vi "PAT Device Software.vi"() -> ()   [LabVIEW 2018]
uses:
  <vilib>/Analysis/baseanly.llb/Mean (DBL).vi
  <vilib>/DAQmx/miscellaneous.llb/DAQmx Fill In Error Info.vi
  <vilib>/DAQmx/read.llb/DAQmx Read (Analog 1D Wfm NChan NSamp).vi
  <vilib>/DAQmx/configure/task.llb/DAQmx Configure Logging (TDMS).vi
  <vilib>/DAQmx/configure/timing.llb/DAQmx Timing (Sample Clock).vi
  <vilib>/DAQmx/create/channels.llb/DAQmx Create Channel (AI-Voltage-Basic).vi
  <vilib>/Instr/_visa.llb/VISA Configure Serial Port (Instr).vi
  <vilib>/Analysis/NI_AALBase.lvlib
panel:
  in  "Relay Comport":refnum<visa-resource-name>="COM7"
  in  "Boolean":bool
  in  "TDMS File Path":path
  in  "Motor Speed Control":dbl=5.0
  in  "Sample Rate":i32=10
  in  "CV2 Input Channel":tag="Dev1/ai0"
  in  "CV1 Input Channel":tag="Dev1/ai1"
  in  "TA Channel":tag="Dev1/ai6"
  in  "RHA Channel":tag="Dev1/ai7"
  in  "P1 Channel":tag="Dev1/ai5"
  out "Stop Test":bool=TRUE
  out "Is PAT Test?":bool=TRUE
  in  "Test Begin":bool
  out "Test Duration":i32
  out "Current Test":string
  out "Test Underway":i32
  out "Number of tests":i32
  out "Test List":i16[](array[numeric])
  out "error out 3":errorcluster
  in  "error in 2":errorcluster
  out "error out 2":errorcluster
  in  "error in":errorcluster
  out "error out":errorcluster
  in  "error in (no error)":errorcluster
  in  "Tab Control":enum32{"PAT Test", "Manual Control"}(tab)
  out "PAT Test Readings":T1 {"B40 S" scale=0.0..100.0; "B15 S" scale=0.0..100.0; "Ex70 S" scale=0.0..100.0; "Ex30 S" scale=0.0..100.0; "In70 S" scale=0.0..100.0; "In30 S" scale=0.0..100.0}
  out "Status":string="Status"
  out "Time":string="Time (s)"
  out "Limit":string="Limit"
  out "Comp":string="Comp"
  out "Units":string="Units"
  out "Measured":string="Measured"
  out "Test Name":string="Test Name"
  out "String 22":string="-0.8"
  out "String 15":string=">="
  out "String 8":string="in H2O"
  out "String":string="Inhalation (30lpm)"
  out "String 24":string="0.8"
  out "String 17":string="<="
  out "String 10":string="in H2O"
  out "String 3":string="Exhalation (30lpm)"
  out "String 23":string="-2.0"
  out "String 16":string=">="
  out "String 9":string="in H2O"
  out "String 2":string="Inhalation (70lpm)"
  out "String 26":string="26"
  out "String 19":string=">="
  out "String 12":string="% O2"
  out "String 5":string="Breathing (15kft)"
  out "String 25":string="2.0"
  out "String 18":string="<="
  out "String 11":string="in H2O"
  out "String 4":string="Exhalation (70lpm)"
  out "String 27":string="89"
  out "String 20":string=">="
  out "String 13":string="% O2"
  out "String 6":string="Breathing (40kft)"
  in  "Start PAT Test":bool
  in  "Stop PAT Test":bool
  out "Test Status:":string
  in  "Results File Location:":path=path "X:/Working/Finn Sowerbutts/Aerox/PAT/CDR Files/PAT Device Software/Test Reports"
  in  "PAT Test Settings":T2={"Test Date:"="", "Test Time:"="", "Pull Test Date:"="", "Operator:"="", "Production Order No.:"="", "Production Lot:"="", "No. Masks in Lot:"="", "Comments:"="", "Array"=[TRUE, TRUE, TRUE, TRUE, TRUE, TRUE], "Test Parameters:"=enum."Quick Test", "Facepiece Leakage"=0.0}
  out "Test Mode:":string[][](table)
  in  "Preset Directory:":path=path "X:/Working/Finn Sowerbutts/Aerox/PAT/CDR Files/PAT Device Software/Presets"
  in  "MC Fields":T3
  in  "MC Instrumentation":T4
  in  "Start Custom Test":bool
  in  "Stop Custom Test":bool
  # "ccm"
  # "s"
  # "Pamb"
  # "Tamb"
  # "Hamb"
  # "in H2O"
  # "°C"
  # "%"
  # "F2"
  # "ccm"
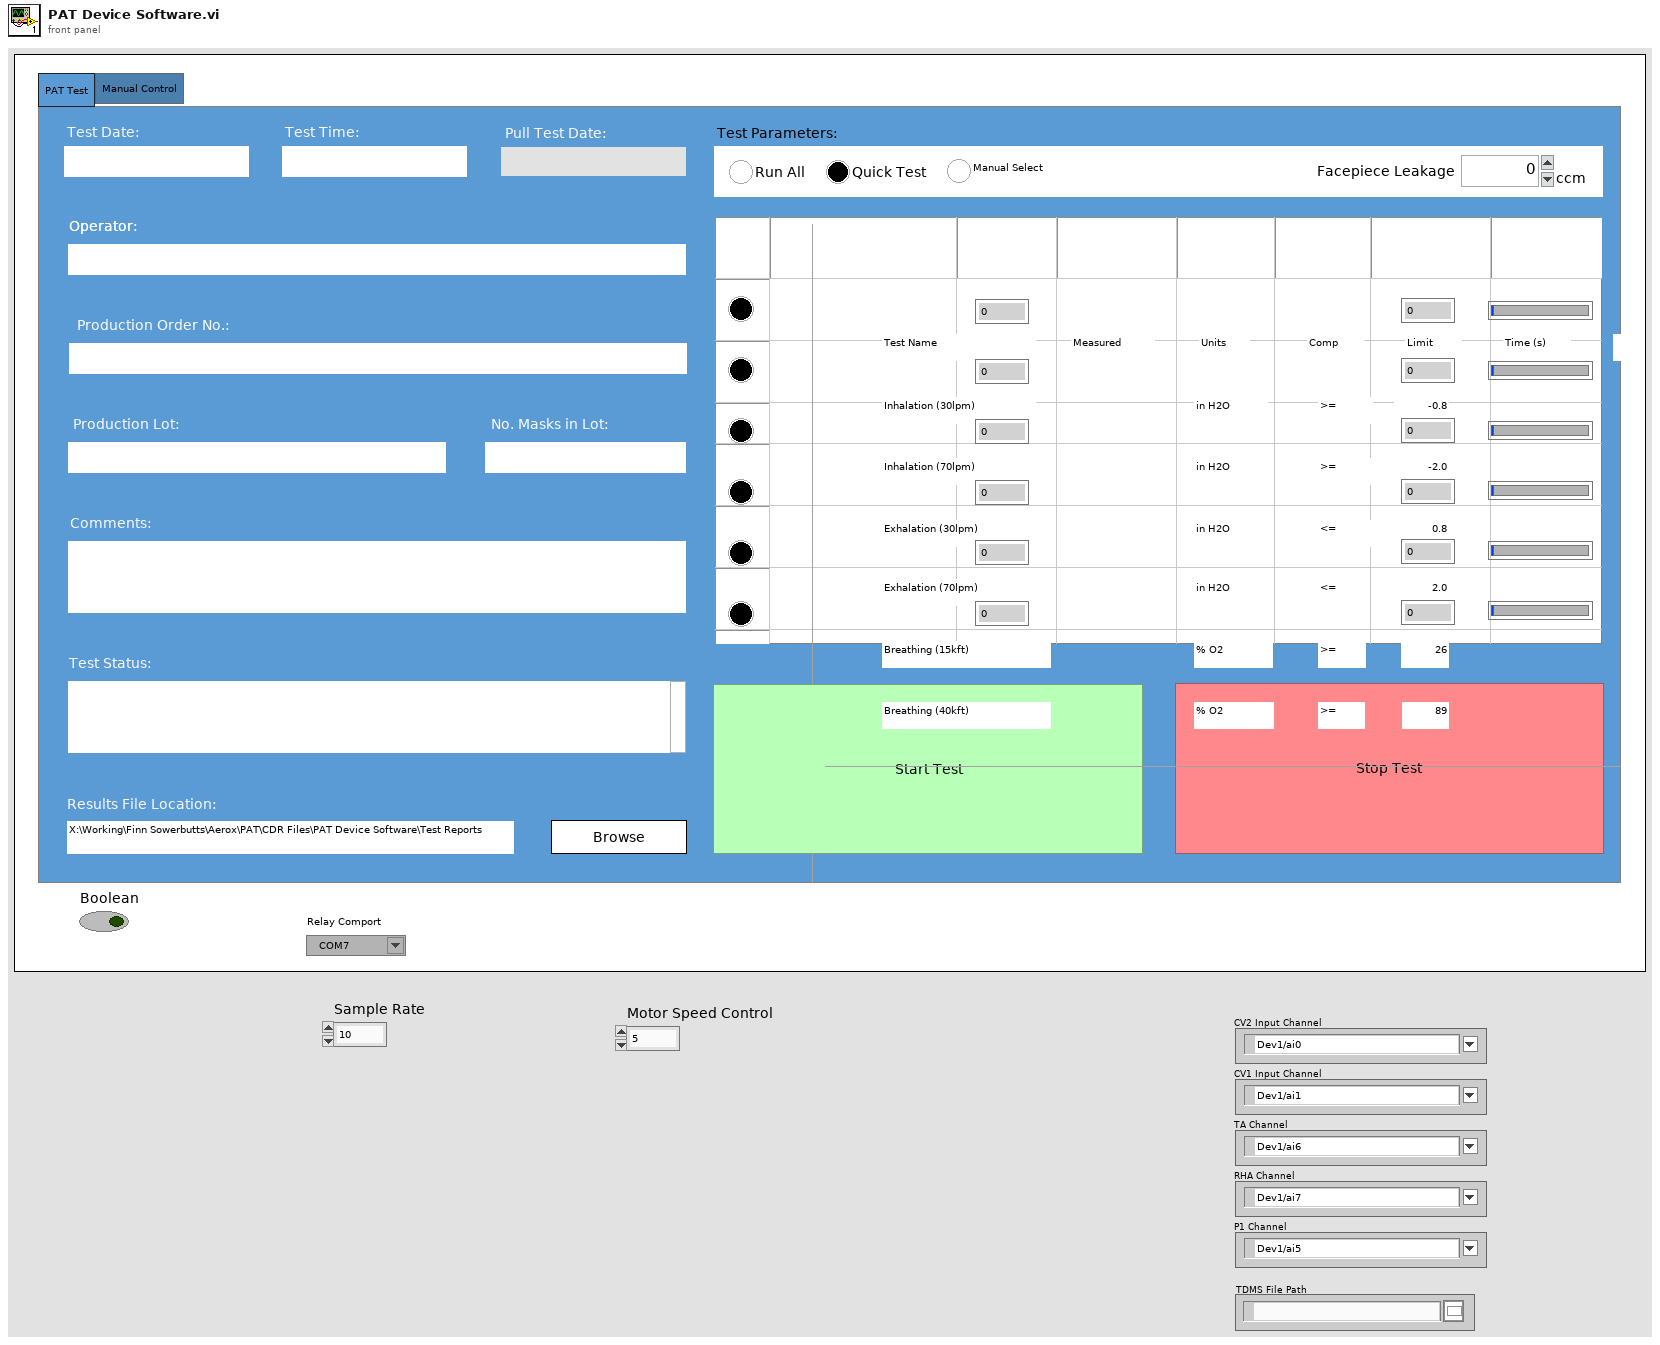
[diagram p1: front panel]
types:
  T1 = cluster{"In30 M":dbl, "In30 T":dbl, "In30 S":u8, "In70 M":dbl, "Ex30 M":dbl, "Ex70 M":dbl, "B40 M":dbl, "B15 M":dbl, "In70 T":dbl, "Ex30 T":dbl, "Ex70 T":dbl, "B40 T":dbl, "B15 T":dbl, "In70 S":u8, "Ex30 S":u8, "Ex70 S":u8, "B15 S":u8, "B40 S":u8}
  T2 = cluster{"Test Date:":string, "Test Time:":string, "Pull Test Date:":string, "Operator:":string, "Production Order No.:":string, "Production Lot:":string, "No. Masks in Lot:":string, "Comments:":string, "Array":bool[], "Test Parameters:":enum32{"Run All", "Quick Test", "Manual Select"}, "Facepiece Leakage":dbl}
  T3 = cluster{"Test Date:":string, "Test Time:":string, "Operator:":string, "PAX Serial No.:":string, "Production Lot:":string, "No. Masks in Lot:":string, "Test Duration":dbl, "Presets in Directory:":i32, "MC Test Length":enum32{"Run Continuously", "Run for:"}, "Current Preset:":string, "Preset Save":bool}
  T4 = cluster{"SV1":bool, "SV2":bool, "SV3":bool, "SV4":bool, "SV5":bool, "SV6":bool, "SV7":bool, "SV8":bool, "SV9":bool, "M1":bool, "MP1":bool, "MP2":bool, "CV1":bool, "CV3":bool, "CV1 Flow Rate:":dbl, "CV2 Flow Rate:":dbl, "P2 Pressure:":dbl, "O2 Concentration:":dbl, "Ambient Pressure:":dbl, "Ambient Temp.:":dbl, "Ambient Humidity:":dbl, "Motor Speed:":dbl, "F2 Leakage":dbl, "P1 Pressure:":dbl}
  T5 = enum8{"Enabled", "Disabled", "Disabled and Grayed Out"}
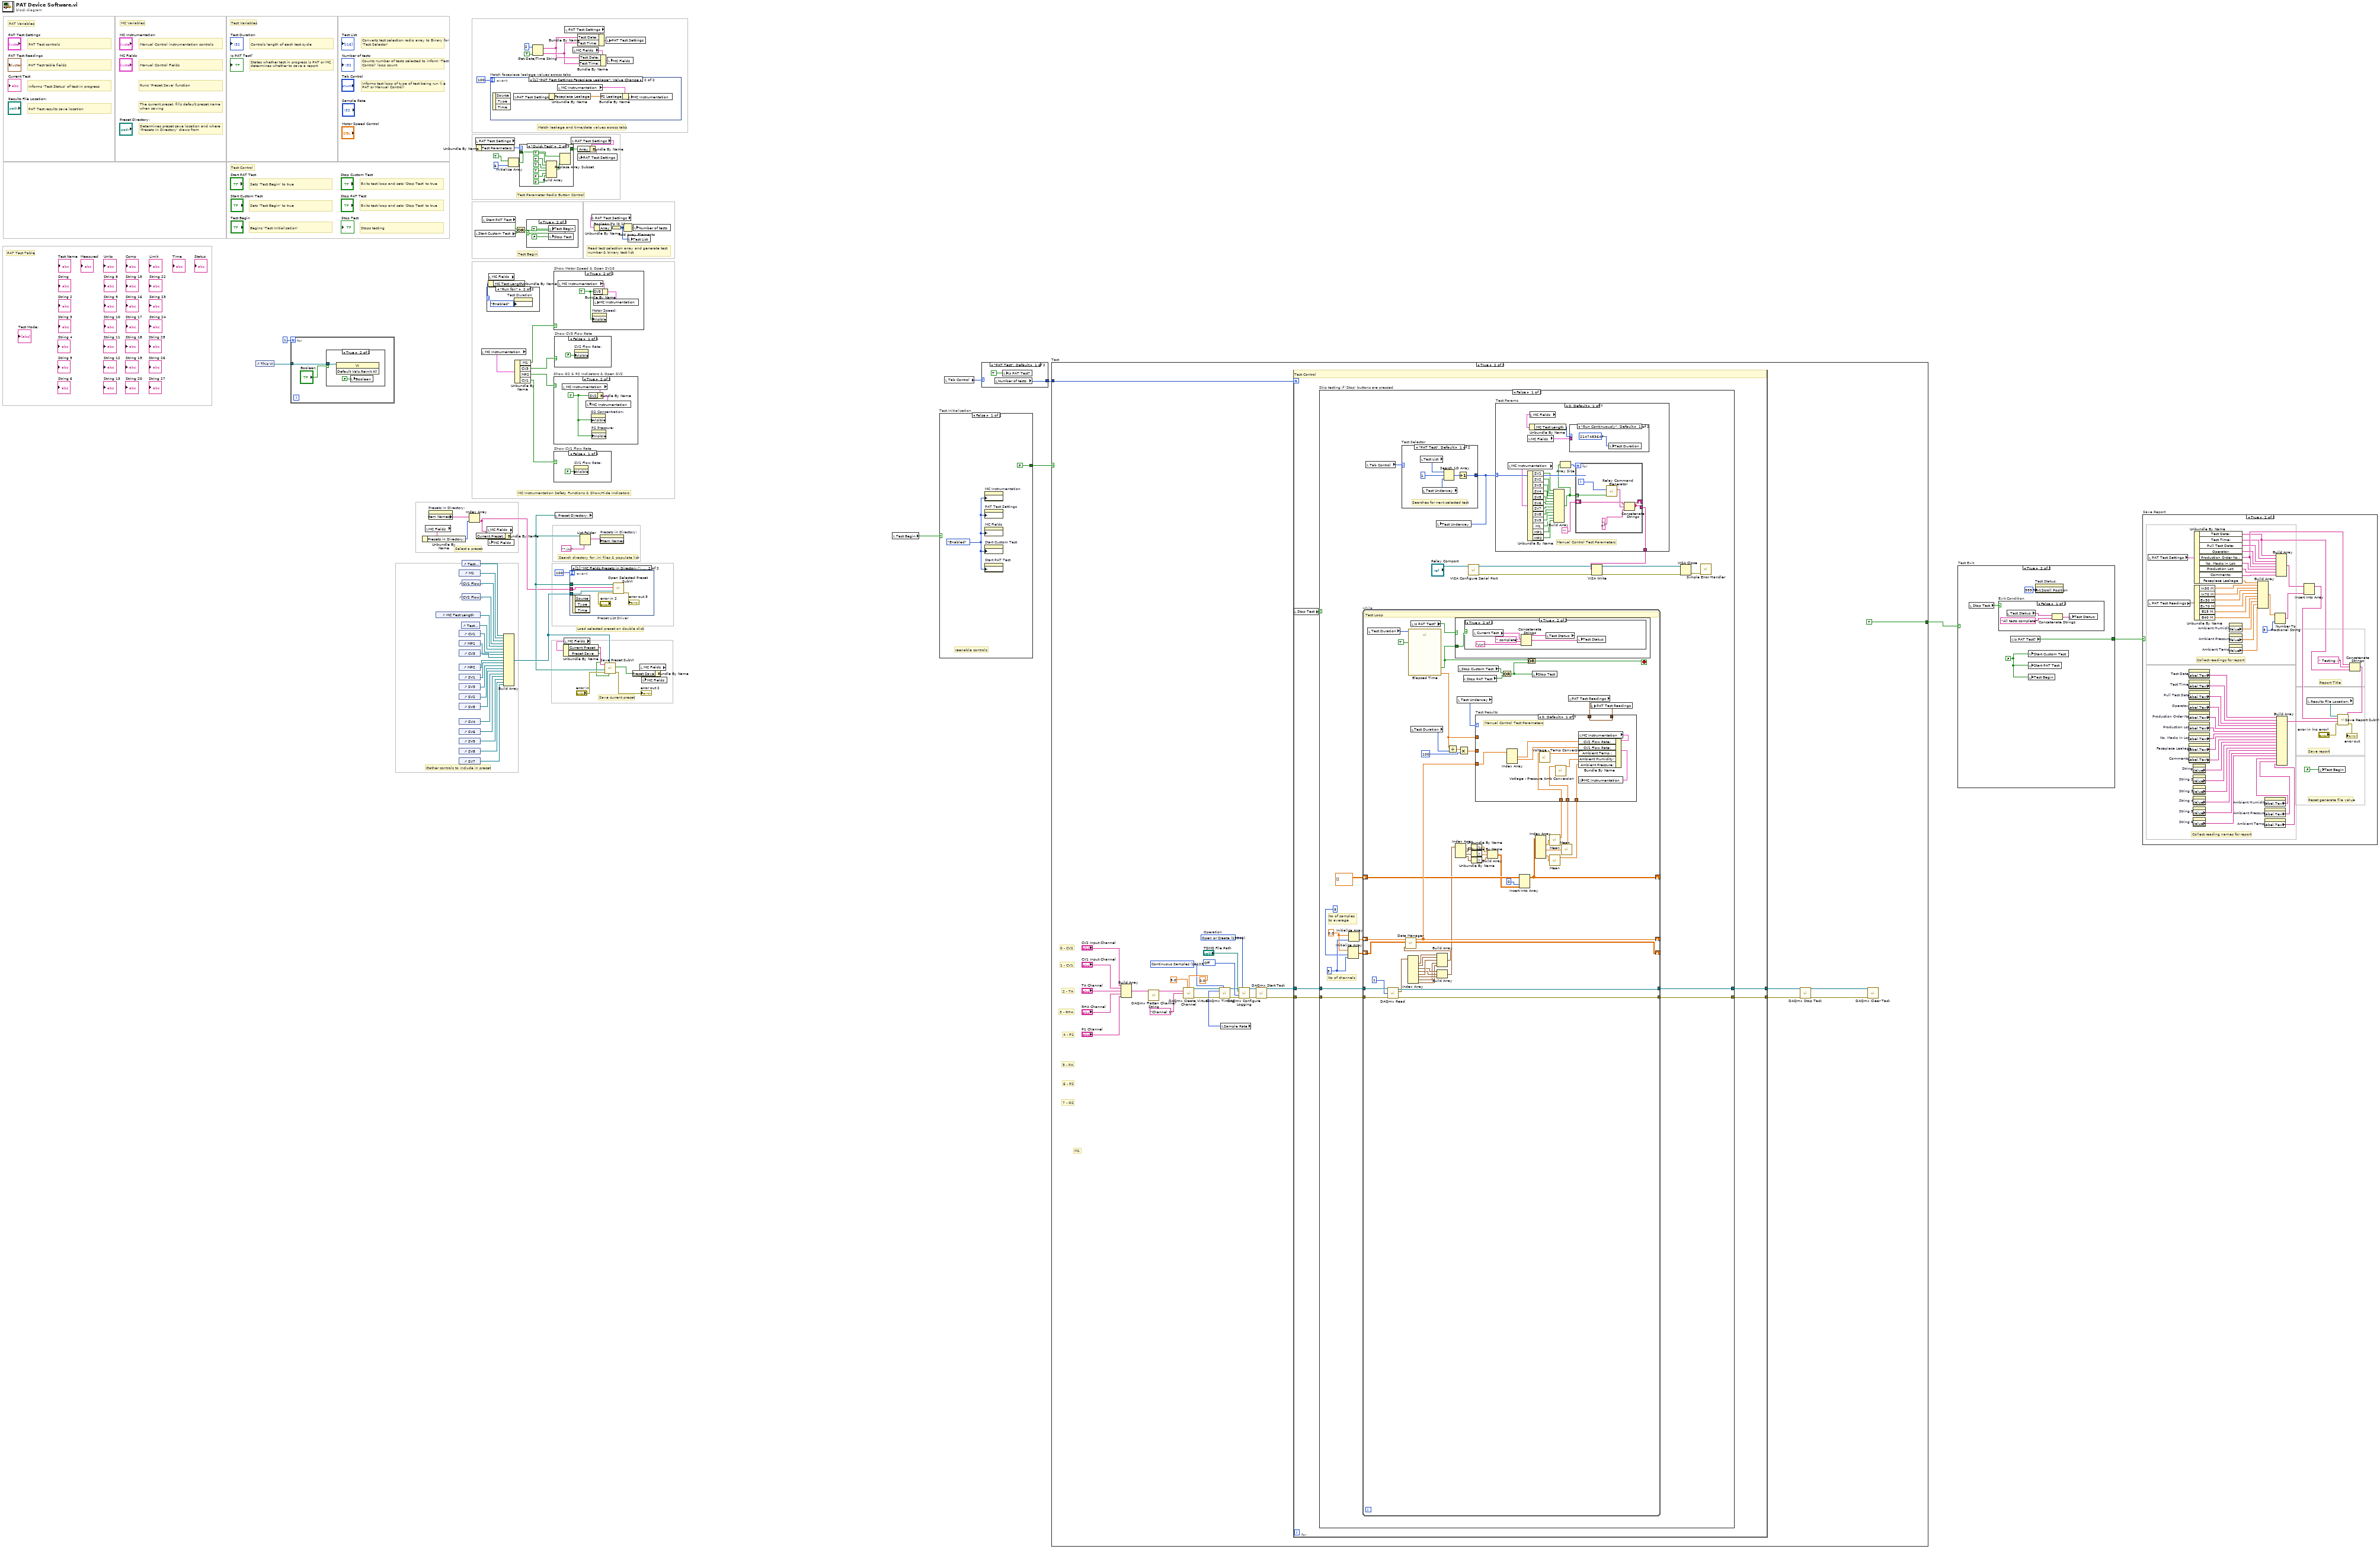
[diagram p0: block diagram]
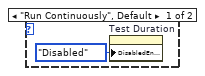
[diagram p2: hidden frame]
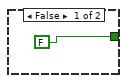
[diagram p4: hidden frame]
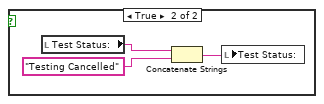
[diagram p5: hidden frame]
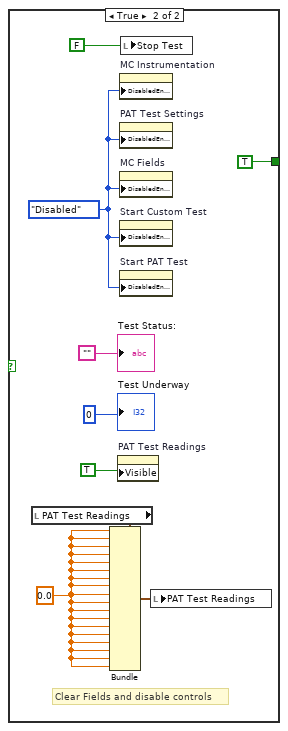
[diagram p6: hidden frame]
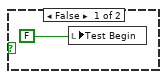
[diagram p7: hidden frame]
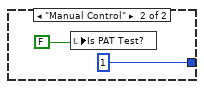
[diagram p8: hidden frame]
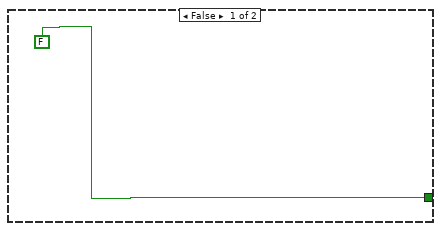
[diagram p9: hidden frame]
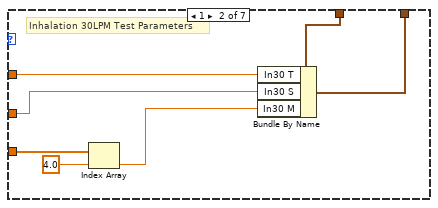
[diagram p12: hidden frame]
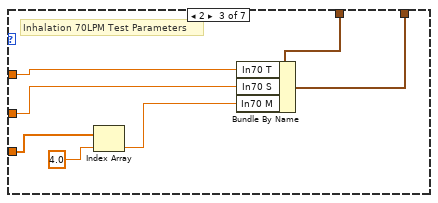
[diagram p13: hidden frame]
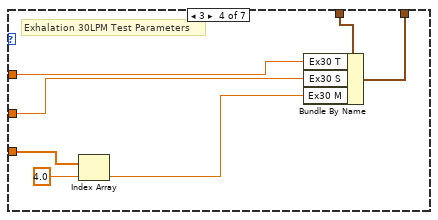
[diagram p14: hidden frame]
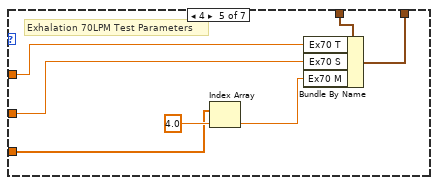
[diagram p15: hidden frame]
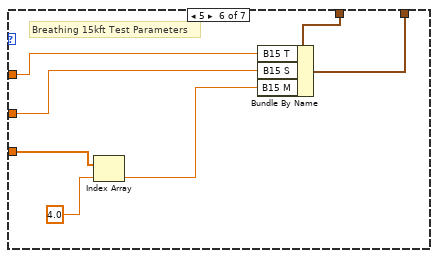
[diagram p16: hidden frame]
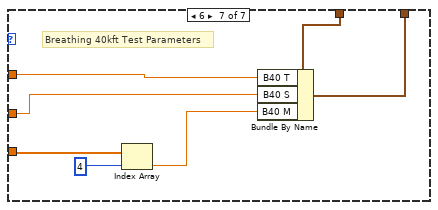
[diagram p17: hidden frame]
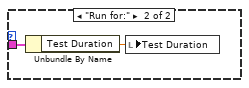
[diagram p18: hidden frame]
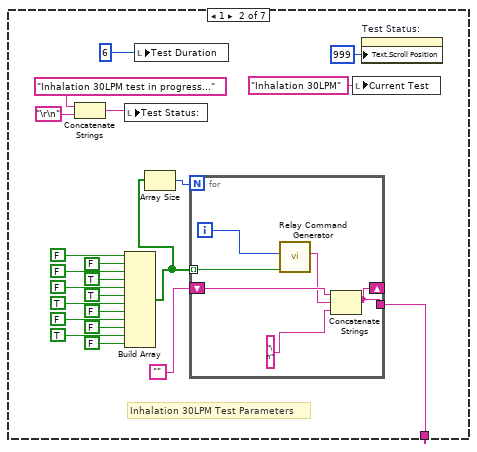
[diagram p19: hidden frame]
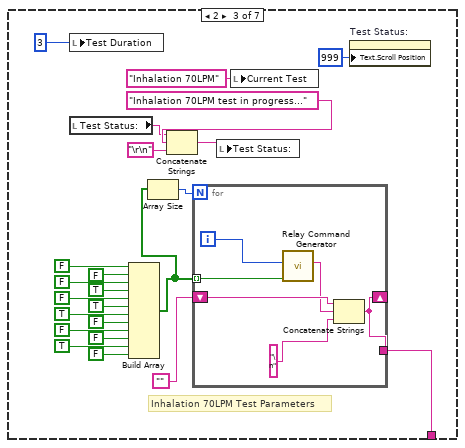
[diagram p20: hidden frame]
diagram:
  # "Save current preset"
  # "Load selected preset on double click"
  # "Search directory for .ini files & populate list"
  # "Gather controls to include in preset"
  # "Select a preset"
  # "Read test selection array and generate test number & binary test list"
  # "MC Instrumentation Safety Functions & Show/Hide Indicators"
  # "Determines preset save location and where 'Presets in Directory' draws from"
  # "Test Control"
  # "Exits test loop and sets 'Stop Test' to true"
  # "Exits test loop and sets 'Stop Test' to true"
  # "Sets 'Test Begin' to true"
  # "Sets 'Test Begin' to true"
  # "The current preset, fills default preset name when saving"
  # "Runs 'Preset Save' function"
  # "PAT Test results save location"
  # "Informs test loop of type of test being run (i.e PAT or Manual Control)"
  # "Counts number of tests selected to inform 'Test Control' loop count"
  # "Stops testing"
  # "Begins 'Test Initialisation'"
  # "States whether test in progress is PAT or MC, determines whether to save a report"
  # "Controls length of each test cycle"
  # "Converts test selection radio array to Binary for 'Test Selector'"
  # "Test Begin"
  # "Test Variables"
  # "Manual Control Fields"
  # "Manual Control instrumentation controls"
  # "PAT Test controls"
  # "PAT Test table fields"
  # "Informs 'Test Status' of test in progress"
  # "MC Variables"
  # "Test Parameter Radio Button Control"
  # "Match leakage and time/date values across tabs"
  # "PAT Variables"
  # "PAT Test Table"
  n1 = control-ref of="This VI"() -> (w12:refnum<vi>)
  n2 = for {
    N: 1 -> [_]
    tunnel: w12 -> [w79]
    n3 = case shown="True" "Boolean" {
      tunnel: w79 -> [_ w81]
      frame False {
      }
      frame True {
        n4 = invoke class="VI" method="Default Vals.Reinit All"(reference=w81) -> ()  [unwired: 2 in, 3 out]
        n5 = local write "Boolean"(FALSE ("Boolean")) -> ()
      }
    }
  }
  n6 = local read "MC Fields"() -> (w32:T3)
  n7 = Unbundle By Name(w32) -> ("Presets in Directory:"=w31:i32)
  n8 = property on="Presets in Directory:" class="LstBox (strict)"() -> ("Item Names"=w54:string[])  [unwired: 2 in, 2 out]
  n9 = control-ref of="MC Test Length"() -> (w34:refnum<vi>)
  n10 = control-ref of="M1"() -> (w71:refnum<vi>)
  n11 = control-ref of="CV1"() -> (w68:refnum<vi>)
  n12 = control-ref of="MP1"() -> (w66:refnum<vi>)
  n13 = control-ref of="CV3"() -> (w67:refnum<vi>)
  n14 = control-ref of="MP2"() -> (w65:refnum<vi>)
  n15 = control-ref of="SV1"() -> (w64:refnum<vi>)
  n16 = control-ref of="SV3"() -> (w63:refnum<vi>)
  n17 = control-ref of="SV2"() -> (w62:refnum<vi>)
  n18 = control-ref of="SV5"() -> (w61:refnum<vi>)
  n19 = control-ref of="SV4"() -> (w60:refnum<vi>)
  n20 = control-ref of="SV6"() -> (w59:refnum<vi>)
  n21 = control-ref of="SV9"() -> (w58:refnum<vi>)
  n22 = control-ref of="SV8"() -> (w57:refnum<vi>)
  n23 = control-ref of="SV7"() -> (w56:refnum<vi>)
  n24 = control-ref of="Test Duration"() -> (w33:refnum<vi>)
  n25 = control-ref of="Test Duration"() -> (w72:refnum<vi>)
  n26 = control-ref of="CV1 Flow Rate:"() -> (w70:refnum<vi>)
  n27 = control-ref of="CV2 Flow Rate:"() -> (w69:refnum<vi>)
  n28 = Index Array(array=w54, index=w31) -> (element=w11:string)
  n29 = local read "Start Custom Test"() -> (w21:bool)
  n30 = local read "PAT Test Settings"() -> (w47:T2)
  n31 = Unbundle By Name(w47) -> ("Test Parameters:"=w43:enum32{"Run All", "Quick Test", "Manual Select"})
  n32 = local read "MC Instrumentation"() -> (w27:T4)
  n33 = local read "Start PAT Test"() -> (w22:bool)
  n34 = local read "MC Fields"() -> (w10:T3)
  n35 = Bundle By Name(cluster=w10, "Current Preset:"=w11) -> (w9:T3)
  n36 = local write "MC Fields"(w9) -> ()
  n37 = local read "MC Fields"() -> (w2:T3)
  n38 = Unbundle By Name(w2) -> ("MC Test Length"=w1:enum32{"Run Continuously", "Run for:"})
  n39 = case shown="\"Run for:\"" w1 {
    frame "Run Continuously", Default {
      n40 = property on="Test Duration" class="DigNum (strict)"("DisabledEnum"=T5."Disabled" ("Disabled")) -> ()  [unwired: 2 in, 2 out]
    }
    frame "Run for:" {
      n41 = property on="Test Duration" class="DigNum (strict)"("DisabledEnum"=T5."Enabled" ("Disabled")) -> ()  [unwired: 2 in, 2 out]
    }
  }
  n42 = event "Match facepiece leakage values across tabs" shown="[1] \"PAT Test Settings.Facepiece Leakage\": Value Change" {
    selector: _ -> [_ _]
    dyn-events: _ -> [_ _]
    timeout: 100 -> [_ _]
    event Timeout {
      n43 = event-data() -> ()  [unwired: 1 in, 3 out]
    }
    event "PAT Test Settings.Facepiece Leakage": Value Change {
      n44 = event-data() -> ()  [unwired: 1 in, 3 out]
      n45 = local read "PAT Test Settings"() -> (w85:T2)
      n46 = Unbundle By Name(w85) -> ("Facepiece Leakage"=w84:dbl)
      n47 = local read "MC Instrumentation"() -> (w86:T4)
      n48 = Bundle By Name(cluster=w86, "F2 Leakage"=w84) -> (w87:T4)
      n49 = local write "MC Instrumentation"(w87) -> ()
    }
  }
  n50 = Build Array(w72, w71, w70, w69, w34, w33, w68, w66, w67, w65, w64, w63, w62, w61, w60, w59, w58, w57, w56) -> (w51:refnum<vi>[])
  n51 = Initialize Array(TRUE, 6) -> (w75:bool[])
  n52 = Unbundle By Name(w27) -> ("M1"=w39:bool, "CV3"=w40:bool, "MP2"=w41:bool, "CV1"=w42:bool)
  n53 = Or(x=w22, y=w21) -> (x .or. y?=w28:bool)
  n54 = case shown="\"Quick Test\"" w43 {
    tunnel: [w88 w91 w100] -> w44
    tunnel: w75 -> [w88 w89 w101]
    frame "Run All", Default {
    }
    frame "Quick Test" {
      n55 = Build Array(TRUE, TRUE, TRUE, TRUE, FALSE, FALSE) -> (w90:bool[])
      n56 = Replace Array Subset(array=w89, new element=w90) -> (w91:bool[])  [unwired: 1 in]
    }
    frame "Manual Select" {
      n57 = local read "PAT Test Settings"() -> (w99:T2)
      n58 = Unbundle By Name(w99) -> ("Array"=w98:bool[])
      n59 = Replace Array Subset(array=w101, new element=w98) -> (w100:bool[])  [unwired: 1 in]
    }
  }
  n60 = case shown="True" w28 {
    frame False {
      n61 = local write "Test Begin"(FALSE) -> ()
    }
    frame True {
      n62 = local write "Test Begin"(TRUE) -> ()
      n63 = local write "Stop Test"(FALSE) -> ()
    }
  }
  n64 = Get Date/Time String(date format (0)=2, want seconds? (F)=TRUE) -> (date string=w30:string, time string=w29:string)  [unwired: 1 in]
  n65 = case "Show O2 & P2 Indicators & Open SV2" shown="True" w41 {
    frame False {
      w105 = FALSE ("Visible")
      n66 = property on="O2 Concentration:" class="DigNum (strict)"("Visible"=w105) -> ()  [unwired: 2 in, 2 out]
      n67 = property on="P2 Pressure:" class="DigNum (strict)"("Visible"=w105) -> ()  [unwired: 2 in, 2 out]
    }
    frame True {
      w106 = TRUE ("Visible")
      n68 = local read "MC Instrumentation"() -> (w108:T4)
      n69 = Bundle By Name(cluster=w108, "SV2"=w106) -> (w107:T4)
      n70 = local write "MC Instrumentation"(w107) -> ()
      n71 = property on="O2 Concentration:" class="DigNum (strict)"("Visible"=w106) -> ()  [unwired: 2 in, 2 out]
      n72 = property on="P2 Pressure:" class="DigNum (strict)"("Visible"=w106) -> ()  [unwired: 2 in, 2 out]
    }
  }
  n73 = case "Show Motor Speed & Open SV10" shown="True" w39 {
    frame False {
      n74 = property on="Motor Speed:" class="DigNum (strict)"("Visible"=FALSE) -> ()  [unwired: 2 in, 2 out]
    }
    frame True {
      w110 = TRUE ("Visible")
      n75 = local read "MC Instrumentation"() -> (w112:T4)
      n76 = property on="Motor Speed:" class="DigNum (strict)"("Visible"=w110) -> ()  [unwired: 2 in, 2 out]
      n77 = Bundle By Name(cluster=w112, "SV5"=w110) -> (w111:T4)
      n78 = local write "MC Instrumentation"(w111) -> ()
    }
  }
  n79 = case "Show CV1 Flow Rate" shown="False" w42 {
    frame False {
      n80 = property on="CV1 Flow Rate:" class="DigNum (strict)"("Visible"=FALSE) -> ()  [unwired: 2 in, 2 out]
    }
    frame True {
      n81 = property on="CV1 Flow Rate:" class="DigNum (strict)"("Visible"=TRUE) -> ()  [unwired: 2 in, 2 out]
    }
  }
  n82 = case "Show CV3 Flow Rate" shown="False" w40 {
    frame False {
      n83 = property on="CV2 Flow Rate:" class="DigNum (strict)"("Visible"=FALSE) -> ()  [unwired: 2 in, 2 out]
    }
    frame True {
      n84 = property on="CV2 Flow Rate:" class="DigNum (strict)"("Visible"=TRUE) -> ()  [unwired: 2 in, 2 out]
    }
  }
  n85 = local read "Preset Directory:"() -> (w15:path)
  n86 = local read "MC Fields"() -> (w8:T3)
  n87 = Unbundle By Name(w8) -> ("Current Preset:"=w7:string, "Preset Save"=w6:bool)
  n88 = local read "PAT Test Settings"() -> (w49:T2)
  n89 = event "Preset List Driver" shown="[1] \"MC Fields.Presets in Directory:\": Double Click" {
    selector: _ -> [_ _]
    dyn-events: _ -> [_ _]
    timeout: 100 -> [_ _]
    tunnel: w11 -> [_ w119]
    tunnel: w15 -> [_ w120]
    tunnel: w51 -> [_ w117]
    event Timeout {
      n90 = event-data() -> ()  [unwired: 1 in, 3 out]
    }
    event "MC Fields.Presets in Directory:": Double Click {
      n91 = event-data() -> ()  [unwired: 1 in, 3 out]
      n92 = call "Open Selected Preset SubVI.vi"("error in (no error)"="error in 2", "Controls"=w117, "Current Preset"=w119, "Preset Directory:"=w120) -> ("error out"=→"error out 3":errorcluster)  [unwired: 7 in]
    }
  }
  n93 = local read "PAT Test Settings"() -> (w46:T2)
  n94 = local read "MC Fields"() -> (w36:T3)
  n95 = Bundle By Name(cluster=w49, "Test Date:"=w30, "Test Time:"=w29) -> (w48:T2)
  n96 = Bundle By Name(cluster=w46, "Array"=w44) -> (w45:T2)
  n97 = local write "PAT Test Settings"(w45) -> ()
  n98 = Bundle By Name(cluster=w36, "Test Date:"=w30, "Test Time:"=w29) -> (w35:T3)
  n99 = List Folder(path=w15, pattern="*.ini") -> (filenames=w53:string[])  [unwired: 2 in, 3 out]
  n100 = local read "PAT Test Settings"() -> (w26:T2)
  n101 = Unbundle By Name(w26) -> ("Array"=w38:bool[])
  n102 = property on="Presets in Directory:" class="LstBox (strict)"("Item Names"=w53) -> ()  [unwired: 2 in, 2 out]
  n103 = call "Save Preset SubVI.vi"("Preset Save"=w6, "Control Settings"=w51, "error in (no error)"="error in", "Preset Directory:"=w15, "Preset Name"=w7) -> ("error out"=→"error out 2":errorcluster, "Reset 'Preset Save'"=w3:bool)  [unwired: 5 in]
  n104 = local write "PAT Test Settings"(w48) -> ()
  n105 = local write "MC Fields"(w35) -> ()
  n106 = Boolean To (0,1)(Boolean=w38) -> (0, 1=w24:i16[])
  n107 = Add Array Elements(numeric array=w24) -> (sum=w25:i16)
  n108 = local write "Test List"(w24) -> ()
  n109 = local write "Number of tests"(w25) -> ()
  n110 = local read "MC Fields"() -> (w4:T3)
  n111 = Bundle By Name(cluster=w4, "Preset Save"=w3) -> (w5:T3)
  n112 = local write "MC Fields"(w5) -> ()
  n113 = local read "Test Begin"() -> (w20:bool)
  n114 = case "Test Initialisation" shown="False" w20 {
    tunnel: [FALSE TRUE] -> w18
    frame False {
      w122 = T5."Enabled" ("Disabled")
      # "reenable controls"
      n115 = property on="MC Instrumentation" class="Clust (strict)"("DisabledEnum"=w122) -> ()  [unwired: 2 in, 2 out]
      n116 = property on="PAT Test Settings" class="Clust (strict)"("DisabledEnum"=w122) -> ()  [unwired: 2 in, 2 out]
      n117 = property on="MC Fields" class="Clust (strict)"("DisabledEnum"=w122) -> ()  [unwired: 2 in, 2 out]
      n118 = property on="Start Custom Test" class="Bool (strict)"("DisabledEnum"=w122) -> ()  [unwired: 2 in, 2 out]
      n119 = property on="Start PAT Test" class="Bool (strict)"("DisabledEnum"=w122) -> ()  [unwired: 2 in, 2 out]
    }
    frame True {
      w125 = 0.0
      w124 = T5."Disabled" ("Disabled")
      # "Clear Fields and disable controls"
      n120 = local read "PAT Test Readings"() -> (w132:T1)
      n121 = Bundle(cluster=w132, "In30 M"=w125, "In30 T"=w125, "In30 S"=w125, "In70 M"=w125, "Ex30 M"=w125, "Ex70 M"=w125, "B40 M"=w125, "B15 M"=w125, "In70 T"=w125, "Ex30 T"=w125, "Ex70 T"=w125, "B40 T"=w125, "B15 T"=w125, "In70 S"=w125, "Ex30 S"=w125, "Ex70 S"=w125, "B15 S"=w125, "B40 S"=w125) -> (w131:T1)
      n122 = property on="PAT Test Readings" class="Clust (strict)"("Visible"=TRUE) -> ()  [unwired: 2 in, 2 out]
      n123 = property on="MC Instrumentation" class="Clust (strict)"("DisabledEnum"=w124) -> ()  [unwired: 2 in, 2 out]
      n124 = property on="PAT Test Settings" class="Clust (strict)"("DisabledEnum"=w124) -> ()  [unwired: 2 in, 2 out]
      n125 = property on="MC Fields" class="Clust (strict)"("DisabledEnum"=w124) -> ()  [unwired: 2 in, 2 out]
      n126 = property on="Start Custom Test" class="Bool (strict)"("DisabledEnum"=w124) -> ()  [unwired: 2 in, 2 out]
      n127 = property on="Start PAT Test" class="Bool (strict)"("DisabledEnum"=w124) -> ()  [unwired: 2 in, 2 out]
      n128 = local write "Stop Test"(FALSE ("Visible")) -> ()
      n129 = local write "PAT Test Readings"(w131) -> ()
      "Test Status:" <- ""
      "Test Underway" <- 0
    }
  }
  n130 = local read "Tab Control"() -> (w23:enum32{"PAT Test", "Manual Control"})
  n131 = case shown="\"PAT Test\", Default" w23 {
    tunnel: [w134 1] -> w37
    frame "PAT Test", Default {
      n132 = local read "Number of tests"() -> (w134:i32)
      n133 = local write "Is PAT Test?"(TRUE ("Boolean")) -> ()
    }
    frame "Manual Control" {
      n134 = local write "Is PAT Test?"(FALSE ("Boolean")) -> ()
    }
  }
  n135 = case "Test" shown="True" w18 {
    tunnel: w37 -> [_ w166]
    tunnel: [FALSE TRUE] -> w19
    frame False {
    }
    frame True {
      w153 = 10231 items=["Off"=10231, "Log and Read"=15842] ("Logging Mode")
      w147 = 10123 items=["Finite Samples"=10178, "Continuous Samples"=10123, "Hardware Timed Single Point"=12522] ("sample mode")
      w152 = 15846 items=["Open"=10437, "Open or Create"=15846, "Create or Replace"=15847, "Create"=15848]  # Operation
      # "M1"
      # "0 - CV2"
      # "1 - CV1"
      # "2 - TA"
      # "3 - RHA"
      # "5 - PA"
      # "6 - P2"
      # "7 - O2"
      # "4 - P1"
      n136 = Build Array("CV2 Input Channel", "CV1 Input Channel", "TA Channel", "RHA Channel", "P1 Channel") -> (w140:tag[])
      n137 = call <vilib>:"DAQmx Flatten Channel String.vi"("names in"=w140) -> ("names out"=w141:string)  [unwired: 13 in, 1 out]
      n138 = call-poly <vilib>:"DAQmx Create Virtual Channel.vi"("maximum value"=5.0, "minimum value"=0.0, "physical channels"=w141, "name to assign"="Channel 1") -> ("task out"=w163:refnum<k21>, "error out"=w164:errorcluster)  [unwired: 10 in]
      n139 = local read "Sample Rate"() -> (w139:i32)
      n140 = call-poly <vilib>:"DAQmx Timing.vi"("task/channels in"=w163, "sample mode"=w147, "rate"=w139, "error in"=w164) -> ("task out"=w149:refnum<k21>, "error out"=w150:errorcluster)  [unwired: 10 in]
      n141 = call-poly <vilib>:"DAQmx Configure Logging.vi"("task/channels in"=w149, "operation"=w152, "file path"="TDMS File Path", "logging mode"=w153, "error in"=w150) -> ("task out"=w148:refnum<k21>, "error out"=w151:errorcluster)  [unwired: 9 in]
      n142 = call <vilib>:"DAQmx Start Task.vi"("task/channels in"=w148, "error in"=w151) -> ("task out"=w155:refnum<k21>, "error out"=w156:errorcluster)  [unwired: 12 in]
      n143 = for {
        N: w166 -> [_]
        tunnel: w155 -> [w170]
        tunnel: w156 -> [w169]
        tunnel: [w168] -> w160
        tunnel: [w167] -> w159
        # "Test Control"
        n144 = local read "Stop Test"() -> (w171:bool)
        n145 = case "Skip testing if 'Stop' buttons are pressed" shown="False" w171 {
          tunnel: w170 -> [w188 w511]
          tunnel: w169 -> [w187 w510]
          tunnel: [w186 w511] -> w168
          tunnel: [w185 w510] -> w167
          frame False {
            w181 = 0.0 ("minimum value")
            w182 = 5
            # "No of samples \nto average"
            # "No of channels"
            n146 = Initialize Array(w181, 5, w182) -> (w184:dbl[][])
            n147 = Initialize Array(w181, w182) -> (w183:dbl[])
            n148 = while {
              tunnel: w188 -> [w227]
              tunnel: w187 -> [w226]
              tunnel: [w224] -> w186
              tunnel: [w225] -> w185
              shift-right: [w219] -> _
              shift-left: w183 -> [w220]
              shift-right: [w221] -> _
              shift-left: w184 -> [w222]
              shift-right: [w209] -> _
              shift-left: dbl[][] [] -> [w211]
              stop <- w241 stop-if-true
              # "Test Loop"
              n149 = local read "Test Duration"() -> (w239:i32)
              n150 = call-poly <vilib>:"DAQmx Read.vi"("task/channels in"=w227, "number of samples per channel"=1, "error in"=w226) -> ("task out"=w224:refnum<k21>, "data"=w191:waveform(dbl)[], "error out"=w225:errorcluster)  [unwired: 10 in]
              n151 = Index Array(array=w191) -> (element #1=w204:waveform(dbl), element #2=w203:waveform(dbl), element #3=w201:waveform(dbl), element #4=w200:waveform(dbl), element #5=w202:waveform(dbl), element #6=w199:waveform(dbl), element #7=w198:waveform(dbl), element #8=w197:waveform(dbl))  [unwired: 8 in]
              n152 = call "Elapsed Time"("Time Target (s)"=w239, "Auto Reset"=TRUE ("Reset")) -> ("Elapsed Time (s)"=w238:dbl, "Time has Elapsed"=w240:bool)  [unwired: 10 in, 6 out]
              n153 = local read "Is PAT Test?"() -> (w218:bool)
              n154 = local read "Test Duration"() -> (w231:i32)
              n155 = Build Array(w204, w203, w202, w198, w197) -> (w195:waveform(dbl)[])
              n156 = call "Data Manager.vi"("Max Av Values In"=w220, "Data Array In"=w222, "Data"=w195) -> ("Max Av Values Out"=w219:dbl[], "Data Array Out"=w221:dbl[][])  [unwired: 6 in]
              n157 = Build Array(w201, w200, w199) -> (w196:waveform(dbl)[])
              n158 = Divide(x=w238, y=w231) -> (x/y=w232:dbl)
              n159 = Index Array(array=w196) -> (element #1=w217:waveform(dbl), element #2=w216:waveform(dbl), element #3=w215:waveform(dbl))  [unwired: 3 in]
              n160 = case shown="True" w218 {
                tunnel: w240 -> [_ w243]
                frame False {
                }
                frame True {
                  n161 = case shown="True" w243 {
                    frame False {
                    }
                    frame True {
                      n162 = local read "Current Test"() -> (w246:string)
                      n163 = local read "Test Status:"() -> (w244:string)
                      n164 = Concatenate Strings(w244, w246, " complete", "\r\n") -> (w245:string)
                      n165 = local write "Test Status:"(w245) -> ()
                    }
                  }
                }
              }
              n166 = local read "Test Underway"() -> (w237:i32)
              n167 = local read "Stop Custom Test"() -> (w235:bool)
              n168 = Multiply(x=w232, y=100) -> (x*y=w229:dbl)
              n169 = local read "Stop PAT Test"() -> (w234:bool)
              n170 = Unbundle By Name(w217) -> ("Y"=w214:dbl[])
              n171 = Unbundle By Name(w216) -> ("Y"=w213:dbl[])
              n172 = Unbundle By Name(w215) -> ("Y"=w212:dbl[])
              n173 = Build Array(w214, w213, w212) -> (w210:dbl[][])
              n174 = Or(x=w235, y=w234) -> (x .or. y?=w236:bool)
              n175 = Insert Into Array(array=w211, index (col)=0, new element=w210) -> (w209:dbl[][])  [unwired: 1 in]
              n176 = Or(x=w240, y=w236) -> (x .or. y?=w241:bool)
              n177 = local write "Stop Test"(w236) -> ()
              n178 = Index Array(array=w209) -> (element #1=w207:dbl[], element #2=w206:dbl[], element #3=w205:dbl[])  [unwired: 6 in]
              n179 = call-poly <vilib>:"Mean.vi"("X"=w207) -> ("mean"=w194:dbl)  [unwired: 1 out]
              n180 = call-poly <vilib>:"Mean.vi"("X"=w205) -> ("mean"=w192:dbl)  [unwired: 1 out]
              n181 = call-poly <vilib>:"Mean.vi"("X"=w206) -> ("mean"=w193:dbl)  [unwired: 1 out]
              n182 = local read "PAT Test Readings"() -> (w233:T1)
              n183 = case "Test Results" shown="0, Default" w237 {
                tunnel: w238 -> [_ w264 w271 w278 w285 w292 w299]
                tunnel: w233 -> [w257 w265 w272 w280 w287 w294 w300]
                tunnel: w229 -> [_ w263 w270 w277 w284 w291 w298]
                tunnel: [w257 w266 w273 w279 w286 w293 w301] -> w228
                tunnel: w219 -> [w256 w261 w268 w275 w281 w288 w295]
                tunnel: w194 -> [w251 _ _ _ _ _ _]
                tunnel: w193 -> [w249 _ _ _ _ _ _]
                tunnel: w192 -> [w253 _ _ _ _ _ _]
                frame 0, Default {
                  # "Manual Control Test Parameters"
                  n184 = Index Array(array=w256) -> (element #1=w255:dbl, element #2=w254:dbl)  [unwired: 3 in, 1 out]
                  n185 = call "Voltage - Temp Conversion.vi"("mean"=w251) -> ("Numeric"=w252:dbl)  [unwired: 10 in]
                  n186 = call "Votlage - Pressure Amb Conversion.vi"("mean"=w249) -> ("Numeric"=w250:dbl)  [unwired: 10 in]
                  n187 = local read "MC Instrumentation"() -> (w259:T4)
                  n188 = Bundle By Name(cluster=w259, "CV2 Flow Rate:"=w255, "CV1 Flow Rate:"=w254, "Ambient Temp.:"=w252, "Ambient Humidity:"=w250, "Ambient Pressure:"=w253) -> (w258:T4)
                  n189 = local write "MC Instrumentation"(w258) -> ()
                }
                frame 1 {
                  # "Inhalation 30LPM Test Parameters"
                  n190 = Index Array(array=w261, index=4.0 ("minimum value")) -> (element=w262:dbl)
                  n191 = Bundle By Name(cluster=w265, "In30 T"=w264, "In30 S"=w263, "In30 M"=w262) -> (w266:T1)
                }
                frame 2 {
                  # "Inhalation 70LPM Test Parameters"
                  n192 = Index Array(array=w268, index=4.0 ("minimum value")) -> (element=w267:dbl)
                  n193 = Bundle By Name(cluster=w272, "In70 T"=w271, "In70 S"=w270, "In70 M"=w267) -> (w273:T1)
                }
                frame 3 {
                  # "Exhalation 30LPM Test Parameters"
                  n194 = Index Array(array=w275, index=4.0 ("minimum value")) -> (element=w274:dbl)
                  n195 = Bundle By Name(cluster=w280, "Ex30 T"=w278, "Ex30 S"=w277, "Ex30 M"=w274) -> (w279:T1)
                }
                frame 4 {
                  # "Exhalation 70LPM Test Parameters"
                  n196 = Index Array(array=w281, index=4.0 ("minimum value")) -> (element=w282:dbl)
                  n197 = Bundle By Name(cluster=w287, "Ex70 T"=w285, "Ex70 S"=w284, "Ex70 M"=w282) -> (w286:T1)
                }
                frame 5 {
                  # "Breathing 15kft Test Parameters"
                  n198 = Index Array(array=w288, index=4.0 ("minimum value")) -> (element=w289:dbl)
                  n199 = Bundle By Name(cluster=w294, "B15 T"=w292, "B15 S"=w291, "B15 M"=w289) -> (w293:T1)
                }
                frame 6 {
                  # "Breathing 40kft Test Parameters"
                  n200 = Index Array(array=w295, index=4) -> (element=w296:dbl)
                  n201 = Bundle By Name(cluster=w300, "B40 T"=w299, "B40 S"=w298, "B40 M"=w296) -> (w301:T1)
                }
              }
              n202 = local write "PAT Test Readings"(w228) -> ()
            }
            n203 = local read "Tab Control"() -> (w190:enum32{"PAT Test", "Manual Control"})
            n204 = case "Test Selector" shown="\"PAT Test\", Default" w190 {
              tunnel: [w504 0] -> w189
              frame "PAT Test", Default {
                # "Searches for next selected test"
                n205 = local read "Test List"() -> (w505:i16[])
                n206 = local read "Test Underway"() -> (w506:i32)
                n207 = Search 1D Array(1D array=w505, element=1, start index (0)=w506) -> (index of element=w508:i32)
                n208 = Increment(x=w508) -> (x+1=w504:i32)
              }
              frame "Manual Control" {
              }
            }
            n209 = local write "Test Underway"(w189) -> ()
            n210 = call-poly "VISA Configure Serial Port"("VISA resource name"="Relay Comport") -> ("VISA resource name out"=w178:refnum<visa-resource-name>, "error out"=w177:errorcluster)  [unwired: 13 in]
            n211 = case "Test Params" shown="0, Default" w189 {
              tunnel: [w302 w331 w359 w388 w417 w446 w475] -> w176
              frame 0, Default {
                # "Manual Control Test Parameters"
                n212 = local read "MC Instrumentation"() -> (w318:T4)
                n213 = local read "MC Fields"() -> (w321:T3)
                n214 = Unbundle By Name(w318) -> ("SV1"=w317:bool, "SV2"=w316:bool, "SV3"=w315:bool, "SV4"=w314:bool, "SV5"=w313:bool, "SV6"=w312:bool, "SV7"=w311:bool, "SV8"=w310:bool, "SV9"=w309:bool, "M1"=w308:bool, "MP1"=w307:bool, "MP2"=w306:bool)
                n215 = local read "MC Fields"() -> (w319:T3)
                n216 = Unbundle By Name(w319) -> ("MC Test Length"=w320:enum32{"Run Continuously", "Run for:"})
                n217 = Build Array(w317, w316, w315, w314, w313, w312, w311, w310, w309, w308, w307, w306) -> (w304:bool[])
                n218 = Array Size(array=w304) -> (size(s)=w305:i32)
                n219 = case shown="\"Run Continuously\", Default" w320 {
                  tunnel: w321 -> [_ w330]
                  frame "Run Continuously", Default {
                    n220 = local write "Test Duration"(2147483647) -> ()
                  }
                  frame "Run for:" {
                    n221 = Unbundle By Name(w330) -> ("Test Duration"=w329:dbl)
                    n222 = local write "Test Duration"(w329) -> ()
                  }
                }
                n223 = for {
                  N: w305 -> [_]
                  tunnel: w304 -> [w326] mode=indexing
                  shift-right: [w323] -> _
                  shift-left: "" -> [w325]
                  tunnel: [w323] -> w302
                  i -> [w327]
                  n224 = call "Relay Command Generator.vi"("Relay"=w327, "On/Off"=w326) -> ("Generated Command"=w324:string)  [unwired: 8 in]
                  n225 = Concatenate Strings(w325, w324, "\n" ("string")) -> (w323:string)
                }
              }
              frame 1 {
                # "Inhalation 30LPM Test Parameters"
                n226 = Concatenate Strings("Inhalation 30LPM test in progress...", "\r\n") -> (w348:string)
                n227 = local write "Test Status:"(w348) -> ()
                n228 = Build Array(FALSE, FALSE ("element"), FALSE ("element"), TRUE ("element"), FALSE ("element"), TRUE ("element"), TRUE ("element"), FALSE ("element"), FALSE ("element"), FALSE ("element"), TRUE ("element"), FALSE ("element")) -> (w345:bool[])
                n229 = local write "Test Duration"(6) -> ()
                n230 = Array Size(array=w345) -> (size(s)=w346:i32)
                n231 = for {
                  N: w346 -> [_]
                  tunnel: w345 -> [w357] mode=indexing
                  shift-right: [w354] -> _
                  shift-left: "" -> [w356]
                  tunnel: [w354] -> w331
                  i -> [w358]
                  n232 = call "Relay Command Generator.vi"("Relay"=w358, "On/Off"=w357) -> ("Generated Command"=w355:string)  [unwired: 8 in]
                  n233 = Concatenate Strings(w356, w355, "\n" ("string")) -> (w354:string)
                }
                n234 = local write "Current Test"("Inhalation 30LPM") -> ()
                n235 = property on="Test Status:" class="Str"("Text.Scroll Position"=999) -> ()  [unwired: 2 in, 2 out]
              }
              frame 2 {
                # "Inhalation 70LPM Test Parameters"
                n236 = local write "Test Duration"(3) -> ()
                n237 = local read "Test Status:"() -> (w375:string)
                n238 = Build Array(FALSE, FALSE ("element"), FALSE ("element"), TRUE ("element"), FALSE ("element"), TRUE ("element"), TRUE ("element"), FALSE ("element"), FALSE ("element"), FALSE ("element"), TRUE ("element"), FALSE ("element")) -> (w374:bool[])
                n239 = Array Size(array=w374) -> (size(s)=w361:i32)
                n240 = Concatenate Strings(w375, "Inhalation 70LPM test in progress...", "\r\n") -> (w381:string)
                n241 = for {
                  N: w361 -> [_]
                  tunnel: w374 -> [w386] mode=indexing
                  shift-right: [w383] -> _
                  shift-left: "" -> [w385]
                  tunnel: [w383] -> w359
                  i -> [w387]
                  n242 = call "Relay Command Generator.vi"("Relay"=w387, "On/Off"=w386) -> ("Generated Command"=w384:string)  [unwired: 8 in]
                  n243 = Concatenate Strings(w385, w384, "\n" ("string")) -> (w383:string)
                }
                n244 = local write "Test Status:"(w381) -> ()
                n245 = local write "Current Test"("Inhalation 70LPM") -> ()
                n246 = property on="Test Status:" class="Str"("Text.Scroll Position"=999) -> ()  [unwired: 2 in, 2 out]
              }
              frame 3 {
                # "Exhalation 30LPM Test Parameters"
                n247 = local write "Test Duration"(8) -> ()
                n248 = local read "Test Status:"() -> (w404:string)
                n249 = Build Array(FALSE, FALSE ("element"), FALSE ("element"), TRUE ("element"), FALSE ("element"), FALSE ("element"), FALSE ("element"), TRUE ("element"), TRUE ("element"), FALSE ("element"), TRUE ("element"), FALSE ("element")) -> (w403:bool[])
                n250 = Array Size(array=w403) -> (size(s)=w390:i32)
                n251 = Concatenate Strings(w404, "Exhalation 30LPM test in progress...", "\r\n") -> (w410:string)
                n252 = for {
                  N: w390 -> [_]
                  tunnel: w403 -> [w415] mode=indexing
                  shift-right: [w412] -> _
                  shift-left: "" -> [w414]
                  tunnel: [w412] -> w388
                  i -> [w416]
                  n253 = call "Relay Command Generator.vi"("Relay"=w416, "On/Off"=w415) -> ("Generated Command"=w413:string)  [unwired: 8 in]
                  n254 = Concatenate Strings(w414, w413, "\n" ("string")) -> (w412:string)
                }
                n255 = local write "Test Status:"(w410) -> ()
                n256 = local write "Current Test"("Exhalation 30LPM") -> ()
                n257 = property on="Test Status:" class="Str"("Text.Scroll Position"=999) -> ()  [unwired: 2 in, 2 out]
              }
              frame 4 {
                # "Exhalation 70LPM Test Parameters"
                n258 = local write "Test Duration"(5) -> ()
                n259 = local read "Test Status:"() -> (w433:string)
                n260 = Build Array(FALSE, FALSE ("element"), FALSE ("element"), TRUE ("element"), FALSE ("element"), FALSE ("element"), FALSE ("element"), TRUE ("element"), TRUE ("element"), FALSE ("element"), TRUE ("element"), FALSE ("element")) -> (w432:bool[])
                n261 = Array Size(array=w432) -> (size(s)=w419:i32)
                n262 = Concatenate Strings(w433, "Exhalation 70LPM test in progress...", "\r\n") -> (w439:string)
                n263 = for {
                  N: w419 -> [_]
                  tunnel: w432 -> [w444] mode=indexing
                  shift-right: [w441] -> _
                  shift-left: "" -> [w443]
                  tunnel: [w441] -> w417
                  i -> [w445]
                  n264 = call "Relay Command Generator.vi"("Relay"=w445, "On/Off"=w444) -> ("Generated Command"=w442:string)  [unwired: 8 in]
                  n265 = Concatenate Strings(w443, w442, "\n" ("string")) -> (w441:string)
                }
                n266 = local write "Test Status:"(w439) -> ()
                n267 = local write "Current Test"("Exhalation 70LPM") -> ()
                n268 = property on="Test Status:" class="Str"("Text.Scroll Position"=999) -> ()  [unwired: 2 in, 2 out]
              }
              frame 5 {
                # "Breathing 15kft Test Parameters"
                n269 = local read "Test Status:"() -> (w462:string)
                n270 = local write "Test Duration"(13) -> ()
                n271 = Build Array(TRUE, TRUE ("element"), TRUE ("element"), TRUE ("element"), TRUE ("element"), FALSE ("element"), FALSE ("element"), FALSE ("element"), FALSE ("element"), TRUE ("element"), FALSE ("element"), TRUE ("element")) -> (w461:bool[])
                n272 = Array Size(array=w461) -> (size(s)=w448:i32)
                n273 = Concatenate Strings(w462, "Breathing 15kft test in progress...", "\r\n") -> (w468:string)
                n274 = for {
                  N: w448 -> [_]
                  tunnel: w461 -> [w473] mode=indexing
                  shift-right: [w470] -> _
                  shift-left: "" -> [w472]
                  tunnel: [w470] -> w446
                  i -> [w474]
                  n275 = call "Relay Command Generator.vi"("Relay"=w474, "On/Off"=w473) -> ("Generated Command"=w471:string)  [unwired: 8 in]
                  n276 = Concatenate Strings(w472, w471, "\n" ("string")) -> (w470:string)
                }
                n277 = local write "Test Status:"(w468) -> ()
                n278 = local write "Current Test"("Breathing 15kft") -> ()
                n279 = property on="Test Status:" class="Str"("Text.Scroll Position"=999) -> ()  [unwired: 2 in, 2 out]
              }
              frame 6 {
                # "Breathing 40kft Test Parameters"
                n280 = local read "Test Status:"() -> (w491:string)
                n281 = local write "Test Duration"(11) -> ()
                n282 = Build Array(TRUE, TRUE ("element"), TRUE ("element"), TRUE ("element"), TRUE ("element"), FALSE ("element"), FALSE ("element"), FALSE ("element"), FALSE ("element"), TRUE ("element"), FALSE ("element"), TRUE ("element")) -> (w490:bool[])
                n283 = Array Size(array=w490) -> (size(s)=w477:i32)
                n284 = Concatenate Strings(w491, "Breathing 40kft test in progress...", "\r\n") -> (w497:string)
                n285 = for {
                  N: w477 -> [_]
                  tunnel: w490 -> [w502] mode=indexing
                  shift-right: [w499] -> _
                  shift-left: "" -> [w501]
                  tunnel: [w499] -> w475
                  i -> [w503]
                  n286 = call "Relay Command Generator.vi"("Relay"=w503, "On/Off"=w502) -> ("Generated Command"=w500:string)  [unwired: 8 in]
                  n287 = Concatenate Strings(w501, w500, "\n" ("string")) -> (w499:string)
                }
                n288 = local write "Test Status:"(w497) -> ()
                n289 = local write "Current Test"("Breathing 40kft") -> ()
                n290 = property on="Test Status:" class="Str"("Text.Scroll Position"=999) -> ()  [unwired: 2 in, 2 out]
              }
            }
            n291 = VISA Write(VISA resource name=w178, write buffer=w176, error in (no error)=w177) -> (VISA resource name out=w174:refnum<visa-resource-name>, error out=w175:errorcluster)  [unwired: 1 out]
            n292 = VISA Close(VISA resource name=w174, error in (no error)=w175) -> (error out=w179:errorcluster)
            n293 = call <vilib>:"Simple Error Handler.vi"("error in (no error)"=w179) -> ()  [unwired: 1 in, 8 out]
          }
          frame True {
          }
        }
      }
      n294 = call <vilib>:"DAQmx Stop Task.vi"("task/channels in"=w160, "error in"=w159) -> ("task out"=w158:refnum<k21>, "error out"=w157:errorcluster)  [unwired: 12 in]
      n295 = call <vilib>:"DAQmx Clear Task.vi"("task in"=w158, "error in"=w157) -> ()  [unwired: 13 in, 1 out]
    }
  }
  n296 = case "Test Exit" shown="True" w19 {
    tunnel: [FALSE w513] -> w14
    frame False {
    }
    frame True {
      w514 = FALSE
      n297 = local read "Stop Test"() -> (w516:bool)
      n298 = case "Exit Condition" shown="False" w516 {
        frame False {
          n299 = local read "Test Status:"() -> (w517:string)
          n300 = Concatenate Strings(w517, "All tests complete") -> (w518:string)
          n301 = local write "Test Status:"(w518) -> ()
        }
        frame True {
          n302 = local read "Test Status:"() -> (w521:string)
          n303 = Concatenate Strings(w521, "Testing Cancelled") -> (w522:string)
          n304 = local write "Test Status:"(w522) -> ()
        }
      }
      n305 = local read "Is PAT Test?"() -> (w513:bool)
      n306 = local write "Start Custom Test"(w514) -> ()
      n307 = local write "Start PAT Test"(w514) -> ()
      n308 = local write "Test Begin"(w514) -> ()
      n309 = property on="Test Status:" class="Str"("Text.Scroll Position"=999) -> ()  [unwired: 2 in, 2 out]
    }
  }
  n310 = case "Save Report" shown="True" w14 {
    frame False {
    }
    frame True {
      # "Reset generate file value"
      # "Save report"
      # "Report Title"
      # "Collect reading names for report"
      # "Collect readings for report"
      n311 = local read "PAT Test Settings"() -> (w551:T2)
      n312 = local read "PAT Test Readings"() -> (w549:T1)
      n313 = property on="Test Date:" class="Str"() -> ("Label.Text"=w564:string)  [unwired: 2 in, 2 out]
      n314 = property on="Test Time:" class="Str"() -> ("Label.Text"=w565:string)  [unwired: 2 in, 2 out]
      n315 = property on="Pull Test Date:" class="Str"() -> ("Label.Text"=w566:string)  [unwired: 2 in, 2 out]
      n316 = property on="Operator:" class="Str"() -> ("Label.Text"=w567:string)  [unwired: 2 in, 2 out]
      n317 = property on="Production Order No.:" class="Str"() -> ("Label.Text"=w568:string)  [unwired: 2 in, 2 out]
      n318 = property on="Production Lot:" class="Str"() -> ("Label.Text"=w569:string)  [unwired: 2 in, 2 out]
      n319 = property on="No. Masks in Lot:" class="Str"() -> ("Label.Text"=w570:string)  [unwired: 2 in, 2 out]
      n320 = property on="Facepiece Leakage" class="DigNum (strict)"() -> ("Label.Text"=w571:string)  [unwired: 2 in, 2 out]
      n321 = property on="Comments:" class="Str"() -> ("Label.Text"=w572:string)  [unwired: 2 in, 2 out]
      n322 = property on="String" class="Str"() -> ("Value"=w548:string)  [unwired: 2 in, 2 out]
      n323 = property on="String 2" class="Str"() -> ("Value"=w547:string)  [unwired: 2 in, 2 out]
      n324 = property on="String 3" class="Str"() -> ("Value"=w546:string)  [unwired: 2 in, 2 out]
      n325 = property on="String 4" class="Str"() -> ("Value"=w545:string)  [unwired: 2 in, 2 out]
      n326 = property on="String 5" class="Str"() -> ("Value"=w544:string)  [unwired: 2 in, 2 out]
      n327 = property on="String 6" class="Str"() -> ("Value"=w543:string)  [unwired: 2 in, 2 out]
      n328 = Unbundle By Name(w551) -> ("Test Date:"=w523:string, "Test Time:"=w525:string, "Pull Test Date:"=w557:string, "Operator:"=w558:string, "Production Order No.:"=w556:string, "No. Masks in Lot:"=w559:string, "Production Lot:"=w560:string, "Comments:"=w561:string, "Facepiece Leakage"=w538:dbl)
      n329 = Unbundle By Name(w549) -> ("In30 M"=w537:dbl, "In70 M"=w536:dbl, "Ex30 M"=w535:dbl, "Ex70 M"=w534:dbl, "B15 M"=w533:dbl, "B40 M"=w532:dbl)
      n330 = property on="Ambient Humidity:" class="DigNum (strict)"() -> ("Value"=w531:dbl)  [unwired: 2 in, 2 out]
      n331 = property on="Ambient Pressure:" class="DigNum (strict)"() -> ("Value"=w530:dbl)  [unwired: 2 in, 2 out]
      n332 = property on="Ambient Temp.:" class="DigNum (strict)"() -> ("Value"=w529:dbl)  [unwired: 2 in, 2 out]
      n333 = Build Array(w538, w537, w536, w535, w534, w533, w532, w531, w530, w529) -> (w539:dbl[])
      n334 = property on="Ambient Humidity:" class="DigNum (strict)"() -> ("Label.Text"=w542:string)  [unwired: 2 in, 2 out]
      n335 = property on="Ambient Pressure:" class="DigNum (strict)"() -> ("Label.Text"=w541:string)  [unwired: 2 in, 2 out]
      n336 = property on="Ambient Temp.:" class="DigNum (strict)"() -> ("Label.Text"=w540:string)  [unwired: 2 in, 2 out]
      n337 = Number To Fractional String(number=w539, precision (6)=3) -> (F-format string=w527:string[])  [unwired: 2 in]
      n338 = Build Array(w523, w525, w557, w558, w556, w559, w560, w561) -> (w528:string[])
      n339 = Build Array(w564, w565, w566, w567, w568, w569, w570, w571, w572, w548, w547, w546, w545, w544, w543, w542, w541, w540) -> (w553:string[])
      n340 = Insert Into Array(array=w528, new element=w527) -> (w524:string[])  [unwired: 1 in]
      n341 = local read "Results File Location:"() -> (w554:path)
      n342 = local write "Test Begin"(FALSE ("Start Custom Test")) -> ()
      n343 = Concatenate Strings(w556, " Testing - ", w523) -> (w552:string)
      n344 = call "Save Report SubVI.vi"("File Name"=w552, "error in (no error)"="error in (no error)", "Value Names"=w553, "Values"=w524, "Results File Location:"=w554) -> ("error out"=→"error out":errorcluster)  [unwired: 6 in]
    }
  }
